vi "Berekenen-b.vi"(6 "K":dbl, 9 "Ti":dbl, 10 "Td":dbl, 11 "T":dbl) -> (2 "B":dbl)   [LabVIEW 2021]
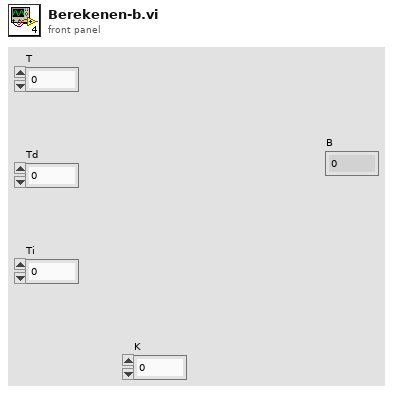
[diagram p1: front panel]
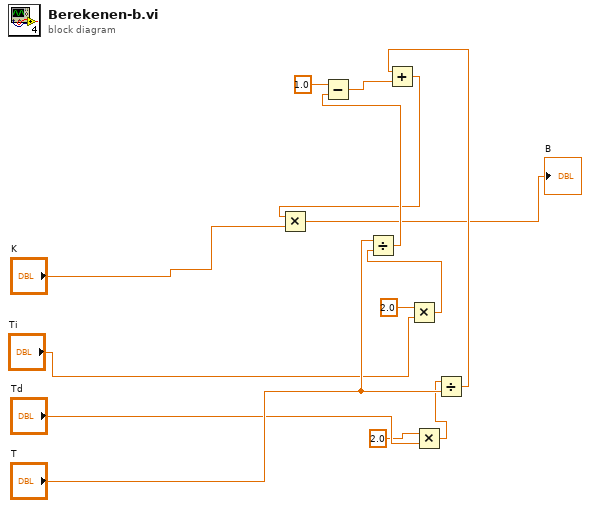
[diagram p0: block diagram]
diagram:
  n1 = Multiply(x=2.0, y="Ti") -> (x*y=w7:dbl)
  n2 = Divide(x="T", y=w7) -> (x/y=w10:dbl)
  n3 = Subtract(x=1.0, y=w10) -> (x-y=w13:dbl)
  n4 = Multiply(x=2.0, y="Td") -> (x*y=w11:dbl)
  n5 = Divide(x=w11, y="T") -> (x/y=w14:dbl)
  n6 = Add(x=w14, y=w13) -> (x+y=w2:dbl)
  n7 = Multiply(x=w2, y="K") -> (x*y=→"B":dbl)
